vi "UI_(01)_Set_startup_controls_state.vi"(3 "error in (no error)":errorcluster, 4 "Settings cluster in":T3={"Defaults"={"Default User"=0.0, "VISA Resource Name "="", "Histogram parameters"={"max"=300.0, "min"=0.0, "# bins"=10, "threshold"=8.0, "thr. type"=enum."higher accepted"}}, "Recording and saving"={"Researcher name"="", "Name prefix"="", "Data post-processing"={"Filter type"=enum."Savitzky-Golay", "Length"=31, "Order"=3}, "Stop at"=0.0, "\"Stop at\" enabled"=FALSE, "Default save folder path"=path "", "Acquisition FPS"=enum."Max"}, "Geometry"={"Sensor board size"=enum."", "Bridge swap"=FALSE, "Twisted neck"=FALSE, "Bridge H. offset"=0.0, "Bridge V. offset"=0.0, "Magnets orientation"=0.0, "Cage type"=0, "Cage parameters"={"Round"=variant(i16 0), "Square"=variant(u16 0), "Donut-maze"=variant(u16 0), "T-maze"=variant(u8 0), "Sociability-maze"=variant(u8 0)}}, "IO parameters"={"IO general config."=0, "IO 1 configuration"=0, "IO 2 configuration"=0, "IO 3 configuration"=0, "IO 4 configuration"=0, "Activate ext. RS-232"=0, "IO inversion config."=0, "Sync capability"=1}, "Conditions presets array"=[{"Enabled"=FALSE, "Name"="", "Specifier(s)"=[], "Response"={"Response type"=enum."Air puff", "TTL port"=enum."Port 1", "TTL pulse length, ms"=0.0}, "Has been set"=FALSE}, {"Enabled"=FALSE, "Name"="", "Specifier(s)"=[], "Response"={"Response type"=enum."Air puff", "TTL port"=enum."Port 1", "TTL pulse length, ms"=0.0}, "Has been set"=FALSE}, {"Enabled"=FALSE, "Name"="", "Specifier(s)"=[], "Response"={"Response type"=enum."Air puff", "TTL port"=enum."Port 1", "TTL pulse length, ms"=0.0}, "Has been set"=FALSE}, {"Enabled"=FALSE, "Name"="", "Specifier(s)"=[], "Response"={"Response type"=enum."Air puff", "TTL port"=enum."Port 1", "TTL pulse length, ms"=0.0}, "Has been set"=FALSE}, {"Enabled"=FALSE, "Name"="", "Specifier(s)"=[], "Response"={"Response type"=enum."Air puff", "TTL port"=enum."Port 1", "TTL pulse length, ms"=0.0}, "Has been set"=FALSE}, {"Enabled"=FALSE, "Name"="", "Specifier(s)"=[], "Response"={"Response type"=enum."Air puff", "TTL port"=enum."Port 1", "TTL pulse length, ms"=0.0}, "Has been set"=FALSE}, {"Enabled"=FALSE, "Name"="", "Specifier(s)"=[], "Response"={"Response type"=enum."Air puff", "TTL port"=enum."Port 1", "TTL pulse length, ms"=0.0}, "Has been set"=FALSE}, {"Enabled"=FALSE, "Name"="", "Specifier(s)"=[], "Response"={"Response type"=enum."Air puff", "TTL port"=enum."Port 1", "TTL pulse length, ms"=0.0}, "Has been set"=FALSE}, {"Enabled"=FALSE, "Name"="", "Specifier(s)"=[], "Response"={"Response type"=enum."Air puff", "TTL port"=enum."Port 1", "TTL pulse length, ms"=0.0}, "Has been set"=FALSE}, {"Enabled"=FALSE, "Name"="", "Specifier(s)"=[], "Response"={"Response type"=enum."Air puff", "TTL port"=enum."Port 1", "TTL pulse length, ms"=0.0}, "Has been set"=FALSE}, {"Enabled"=FALSE, "Name"="", "Specifier(s)"=[], "Response"={"Response type"=enum."Air puff", "TTL port"=enum."Port 1", "TTL pulse length, ms"=0.0}, "Has been set"=FALSE}, {"Enabled"=FALSE, "Name"="", "Specifier(s)"=[], "Response"={"Response type"=enum."Air puff", "TTL port"=enum."Port 1", "TTL pulse length, ms"=0.0}, "Has been set"=FALSE}, {"Enabled"=FALSE, "Name"="", "Specifier(s)"=[], "Response"={"Response type"=enum."Air puff", "TTL port"=enum."Port 1", "TTL pulse length, ms"=0.0}, "Has been set"=FALSE}, {"Enabled"=FALSE, "Name"="", "Specifier(s)"=[], "Response"={"Response type"=enum."Air puff", "TTL port"=enum."Port 1", "TTL pulse length, ms"=0.0}, "Has been set"=FALSE}], "Calibration parameters"={"Timing calibration sw/hw"=1.0, "True FPS"=80.0, "True frame time, s"=80.0, "Disp. calibration info"=[]}} {"Calibration parameters"."True frame time, s" format="%.10g"; "Calibration parameters"."Disp. calibration info"."Speed, µl per ms" format="%.3g"; "Calibration parameters"."True FPS" format="%.10g"; "Calibration parameters"."Timing calibration sw/hw" format="%.10g"; "Conditions presets array"."Specifier(s)"."Validity criteria(s)"."Validity value" min=0.0 step=0.1 format="%.2g"; "Conditions presets array"."Specifier(s)"."Value" step=1.0 format="%#.2g"; "Recording and saving"."Data post-processing"."Order" min=3 max=11 step=2; "Recording and saving"."Data post-processing"."Length" min=5 max=301 step=2; "Geometry"."Cage type" items=["Round", "Square", "Donut-maze", "T-maze", "Sociability maze", ""]}, 5 "All UI references in":T24) -> (0 "error out":errorcluster)   [LabVIEW 2018, in "Tracker Main.lvlib"]
uses:
  Tracker Main.lvlib
  Common/Typedefs/CTL_All_UI_References_2.ctl
  Common/Typedefs/CTL_Panes_and_VIs_References.ctl
  Common/Typedefs/CTL_Indicators_References_2.ctl
  Common/Typedefs/CTL_Controls_References_2.ctl
  SubVi's/Controls/CTL_Histogram_Properties.ctl
  <vilib>/Utility/miscctls.llb/LVRangeTypeDef.ctl
  Common/Typedefs/CTL_Settings_cluster_2.ctl
  SubVi's/Controls/CTL_Histogram_parameters.ctl
  SubVi's/Controls/CTL_Filter_selector.ctl
  SubVi's/Controls/CTL_Acquisition_speed_selector.ctl
  Common/Typedefs/CTL_Segmented_plot_parameters_2.ctl
  Cage Diagram/Typedefs/CTL_Cage_type.ctl
  SubVi's/Controls/CTL_Cage_all_segmentation_params_set.ctl
  SubVi's/Controls/CTL_IO_params_cluster.ctl
  SubVi's/Controls/CTL_Conditions_Array.ctl
  SubVi's/Controls/CTL_Conditions_Cluster.ctl
  SubVi's/Controls/CTL_Condition_type.ctl
  SubVi's/Controls/CTL_Comparison_type.ctl
  SubVi's/Controls/CTL_Validity_check_criteria.ctl
  SubVi's/Controls/CTL_Response_info.ctl
  SubVi's/Controls/CTL_Condition_response_type.ctl
  SubVi's/Controls/CTL_Reponse_port_info.ctl
  SubVi's/Controls/CTL_Calibration_parameters.ctl
  SubVi's/Controls/CTL_Dispenser_calibration_info.ctl
  <vilib>/Utility/miscctls.llb/LVPointTypeDef.ctl
  Common/Typedefs/CTL_IO_Ports_activity_indicator.ctl
  <vilib>/Utility/error.llb/Error Cluster From Error Code.vi
  <vilib>/ErrorRing/Error Ring.xnode
  Common_Resources.lvlib
  Cage Diagram/Cage Diagram.lvlib
panel:
  out "Controls References":T1
  out "Indicators References":T2
  in  "Histogram initialization cluster":T21={"X Scale.Range"={"Minimum"=0.0, "Maximum"=13.0, "Increment"=1.0, "Minor Increment"=1.0, "Start"=0.0}, "Caption.Text"="Zone preference (normalized)", "X Scale.Offset and Multiplier:Multiplier"=1.0, "X Scale.Offset and Multiplier:Offset"=0.0, "X Scale.Scale Fit"=2, "X Scale.Display Format:Precision"=0, "Y Scale.Mapping Mode"=0, "Zones preference empty initialized array"=[0, 0, 0, 0, 0, 0, 0, 0, 0, 0, 0, 0, 0, 0], "Plot.Fill/Point Color"=15790320}
  out "Panes references":T23
  out "Controls references params":string[][](array[string])
  out "Indicators references params":string[][](array[string])
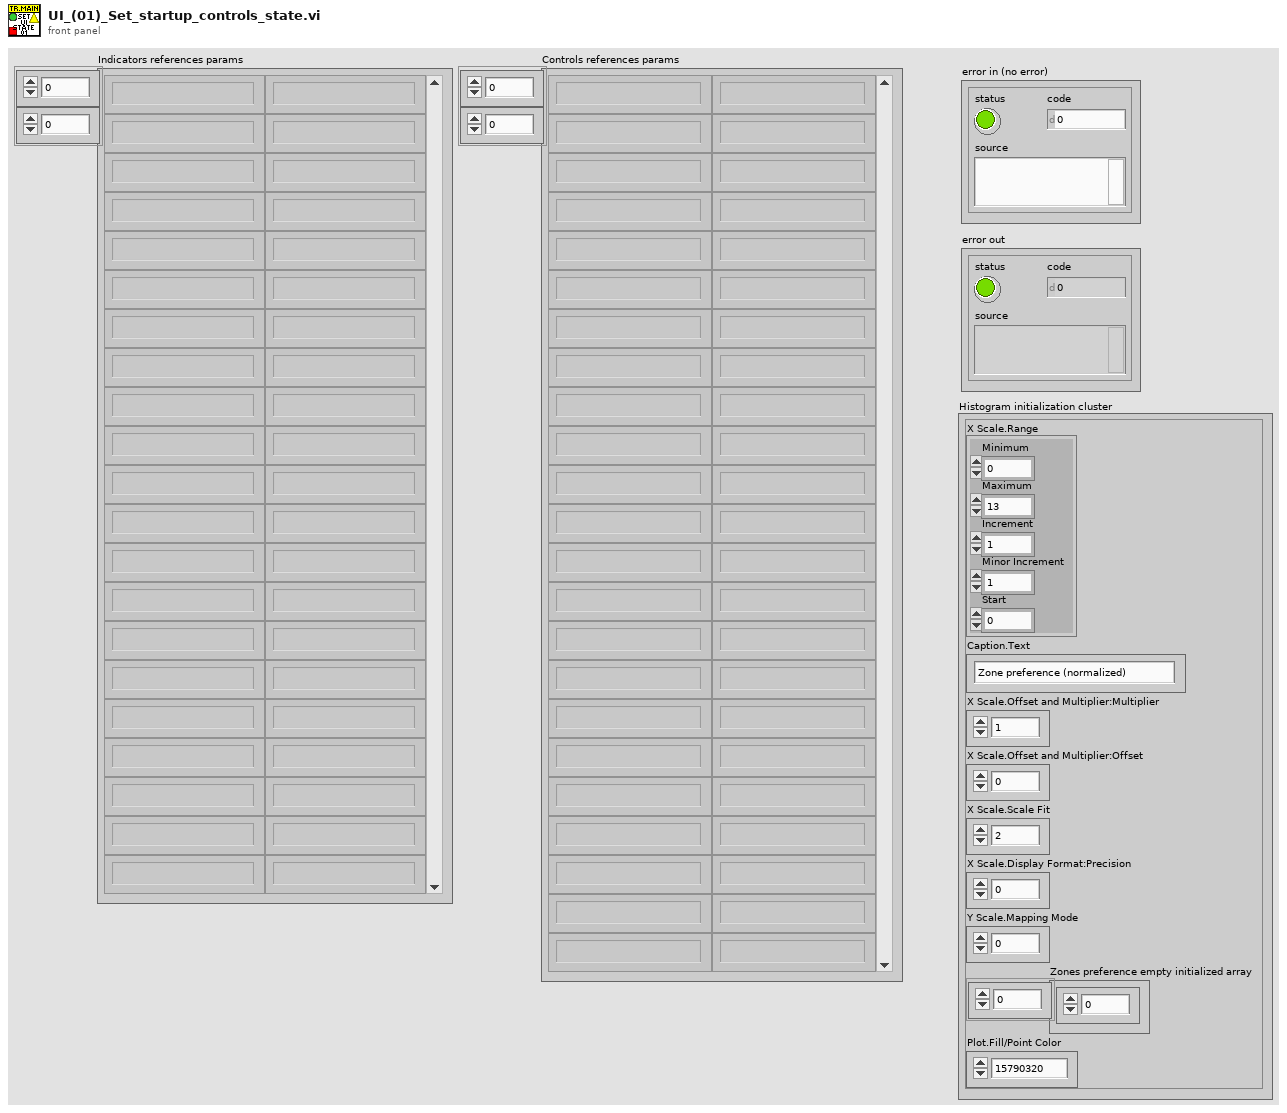
[diagram p1: front panel]
types:
  T1 = typedef "Common_Resources.lvlib/CTL_Controls_References_2.ctl" = cluster{"Timeline":refnum<vi>, "Play/Pause":refnum<vi>, "Record/Stop":refnum<vi>, "Exact time pos.":refnum<vi>, "Add Reward":refnum<vi>, "Modify Reward":refnum<vi>, "Remove Reward":refnum<vi>, "Show zones":refnum<vi>, "Show magnets":refnum<vi>, "Rainbow (time)":refnum<vi>, "Rainbow (speed)":refnum<vi>, "Show heatmap":refnum<vi>, "Show full track":refnum<vi>, "Playback speed":refnum<vi>, "Trace, s":refnum<vi>, "Set/Rec and Analyse Tab":refnum<vi>, "Reward and stimulation":refnum<vi>, "Speed threshold":refnum<vi>, "Multiplyer of chart RX":refnum<vi>, "Reset barplot":refnum<vi>, "Open File":refnum<vi>, "Start over":refnum<vi>}
  T2 = typedef "Common_Resources.lvlib/CTL_Indicators_References_2.ctl" = cluster{"HW info":refnum<vi>, "Port":refnum<vi>, "Cage size":refnum<vi>, "Current zone":refnum<vi>, "Current Time":refnum<vi>, "Since track start":refnum<vi>, "Key_pressed":refnum<vi>, "Status":refnum<vi>, "Status History":refnum<vi>, "IO status":refnum<vi>, "Ports Activity":refnum<vi>, "Active rules":refnum<vi>, "Histograms":refnum<vi>, "Mouse speed":refnum<vi>, "Mouse speed, mm/s":refnum<vi>, "Average speed, mm/s":refnum<vi>, "Run distance, m":refnum<vi>, "Running, perc. of time":refnum<vi>, "CPU load":refnum<vi>, "Diagram ref":refnum<vi>}
  T3 = typedef "Common_Resources.lvlib/CTL_Settings_cluster_2.ctl" = cluster{"Defaults":cluster{"Default User":dbl, "VISA Resource Name ":string, "Histogram parameters":T4}, "Recording and saving":cluster{"Researcher name":string, "Name prefix":string, "Data post-processing":T5, "Stop at":dbl, "\"Stop at\" enabled":bool, "Default save folder path":path, "Acquisition FPS":T6}, "Geometry":T7, "IO parameters":T10, "Conditions presets array":T11, "Calibration parameters":T19}
  T4 = typedef "Common_Resources.lvlib/CTL_Histogram_parameters.ctl" = cluster{"max":dbl, "min":dbl, "# bins":i32, "threshold":dbl, "thr. type":enum16{"higher accepted", "lower accepted"}}
  T5 = typedef "Common_Resources.lvlib/CTL_Filter_selector.ctl" = cluster{"Filter type":enum16{"None", "Savitzky-Golay"}, "Length":i32, "Order":i32}
  T6 = typedef "Common_Resources.lvlib/CTL_Acquisition_speed_selector.ctl" = enum16{"Max", "Optimal", "Eco"}
  T7 = typedef "Common_Resources.lvlib/CTL_Segmented_plot_parameters_2.ctl" = cluster{"Sensor board size":enum16{"", "Large"}, "Bridge swap":bool, "Twisted neck":bool, "Bridge H. offset":sgl, "Bridge V. offset":sgl, "Magnets orientation":sgl, "Cage type":T8, "Cage parameters":T9}
  T8 = typedef "Cage Diagram.lvlib/CTL_Cage_type.ctl" = u16
  T9 = typedef "Common_Resources.lvlib/CTL_Cage_all_segmentation_params_set.ctl" = cluster{"Round":variant, "Square":variant, "Donut-maze":variant, "T-maze":variant, "Sociability-maze":variant}
  T10 = typedef "Common_Resources.lvlib/CTL_IO_params_cluster.ctl" = cluster{"IO general config.":u16, "IO 1 configuration":u16, "IO 2 configuration":u16, "IO 3 configuration":u16, "IO 4 configuration":u16, "Activate ext. RS-232":u16, "IO inversion config.":u16, "Sync capability":u8}
  T11 = typedef "Common_Resources.lvlib/CTL_Conditions_Array.ctl" = T12[]
  T12 = typedef "Common_Resources.lvlib/CTL_Conditions_Cluster.ctl" = cluster{"Enabled":bool, "Name":string, "Specifier(s)":cluster{"Specifier enabled":bool, "Condition type":T13, "Comparison type":T14, "Value":dbl, "Validity criteria(s)":cluster{"V. check enabled":bool, "Criteria":T15, "Validity value":dbl}[]}[], "Response":T16, "Has been set":bool}
  T13 = typedef "Common_Resources.lvlib/CTL_Condition_type.ctl" = enum16{"Speed", "Zone", "Angle to wall"}
  T14 = typedef "Common_Resources.lvlib/CTL_Comparison_type.ctl" = enum16{"Less", "Less or Equal", "Equal", "Greater or Equal", "Greater", "Not Equal"}
  T15 = typedef "Common_Resources.lvlib/CTL_Validity_check_criteria.ctl" = enum16{"Running bout (seconds)", "Running bout (meters)"}
  T16 = typedef "Common_Resources.lvlib/CTL_Response_info.ctl" = cluster{"Response type":T17, "TTL port":T18, "TTL pulse length, ms":dbl}
  T17 = typedef "Common_Resources.lvlib/CTL_Condition_response_type.ctl" = enum16{"None", "Air puff", "Liquid reward", "TTL pulse", "TTL pulse (ubr)", "TTL signal"}
  T18 = typedef "Common_Resources.lvlib/CTL_Reponse_port_info.ctl" = enum16{"Port 1", "Port 2", "Port 3", "Port 4"}
  T19 = typedef "Common_Resources.lvlib/CTL_Calibration_parameters.ctl" = cluster{"Timing calibration sw/hw":dbl, "True FPS":dbl, "True frame time, s":dbl, "Disp. calibration info":T20}
  T20 = typedef "Common_Resources.lvlib/CTL_Dispenser_calibration_info.ctl" = cluster{"Channel":u8, "Speed, µl per ms":dbl}[]
  T21 = typedef "Common_Resources.lvlib/CTL_Histogram_Properties.ctl" = cluster{"X Scale.Range":T22, "Caption.Text":string, "X Scale.Offset and Multiplier:Multiplier":dbl, "X Scale.Offset and Multiplier:Offset":dbl, "X Scale.Scale Fit":u8, "X Scale.Display Format:Precision":u8, "Y Scale.Mapping Mode":u8, "Zones preference empty initialized array":i32[], "Plot.Fill/Point Color":u32}
  T22 = typedef "LVRangeTypeDef.ctl" = cluster{"Minimum":dbl, "Maximum":dbl, "Increment":dbl, "Minor Increment":dbl, "Start":dbl}
  T23 = typedef "Common_Resources.lvlib/CTL_Panes_and_VIs_References.ctl" = cluster{"Pane":refnum<vi>, "This VI":refnum<vi>, "Menu":refnum<k9>}
  T24 = typedef "Common_Resources.lvlib/CTL_All_UI_References_2.ctl" = cluster{"Service references":T23, "Indicators References":T2, "Controls References":T1}
  T25 = typedef "LVPointTypeDef.ctl" = cluster{"Horizontal":i16, "Vertical":i16}
  T26 = typedef "Common_Resources.lvlib/CTL_IO_Ports_activity_indicator.ctl" = cluster{"IO1 act":bool, "IO2 act":bool, "IO3 act":bool, "IO4 act":bool}
  T27 = cluster{"01":bool, "02":bool, "03":bool, "04":bool, "05":bool, "06":bool, "07":bool, "08":bool, "09":bool}
  T28 = enum8{"Enabled", "Disabled", "Disabled and Grayed Out"}
  T29 = enum32{"Page Enabled", "Page Disabled", "Page Disabled & Grayed"}
  T30 = cluster{"Slider":dbl, "Slider":dbl, "Slider":dbl}
  T31 = typedef "Common_Resources.lvlib/CTL_IO_status_indicator_2.ctl" = cluster{"IO1":bool, "IO2":bool, "IO3":bool, "IO4":bool, "St1":bool, "St2":bool, "St3":bool, "St4":bool, "Ext1":bool, "Ext2":bool, "Ext3":bool, "Ext4":bool, "Syn1":bool, "Syn2":bool, "Syn3":bool, "Syn4":bool}
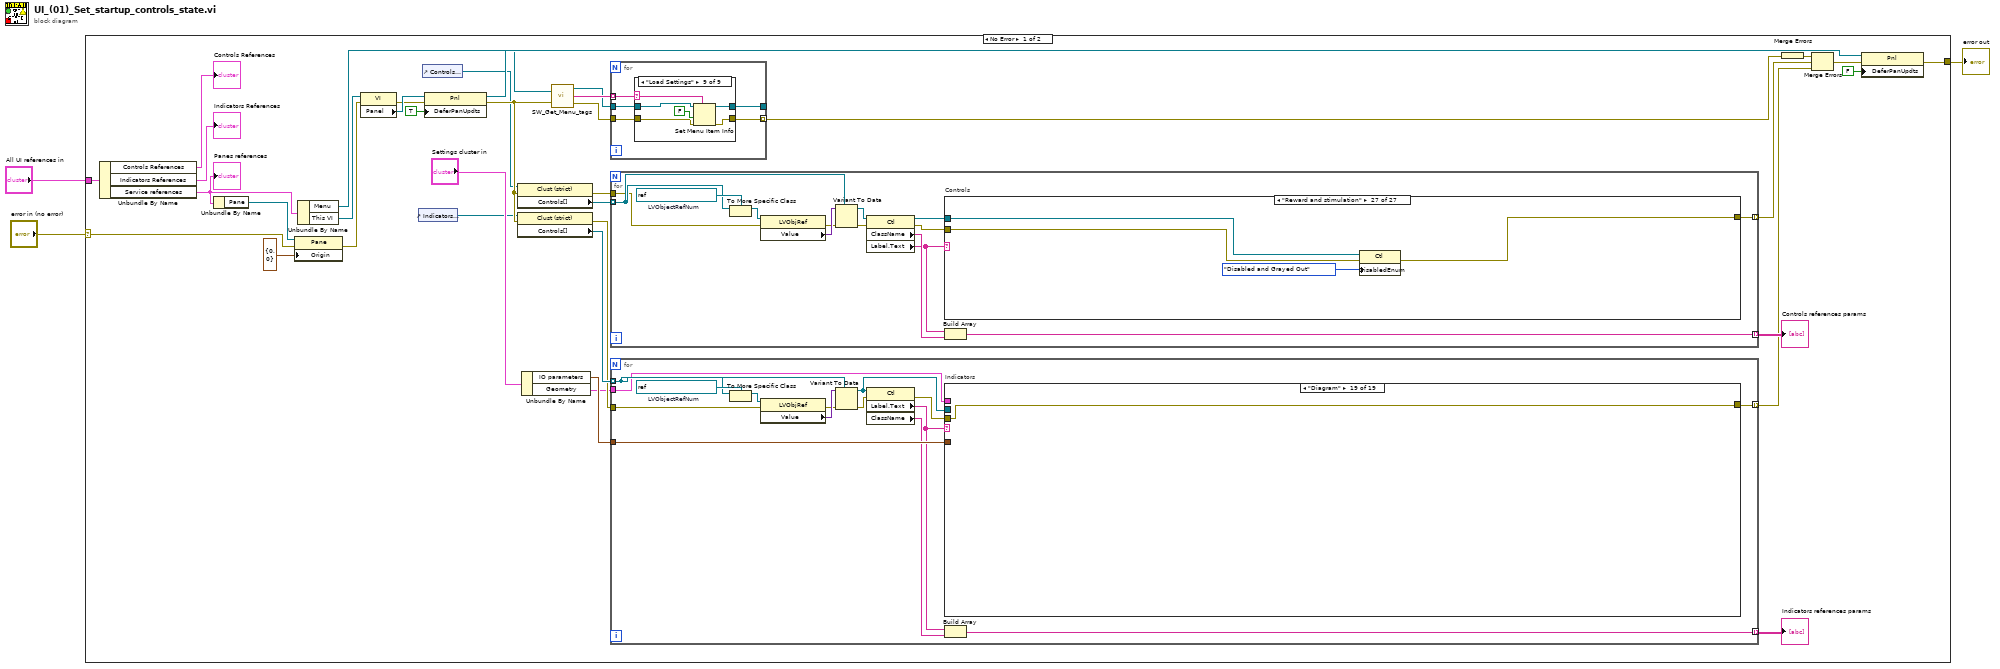
[diagram p0: block diagram]
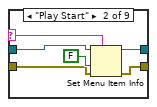
[diagram p3: hidden frame]
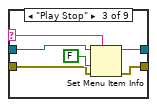
[diagram p4: hidden frame]
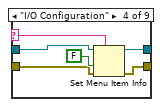
[diagram p5: hidden frame]
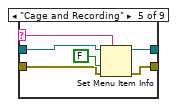
[diagram p6: hidden frame]
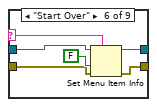
[diagram p7: hidden frame]
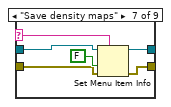
[diagram p8: hidden frame]
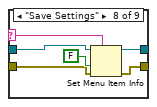
[diagram p9: hidden frame]
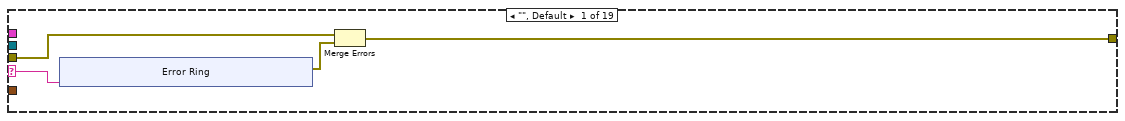
[diagram p10: hidden frame]
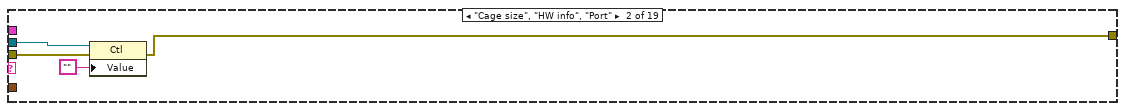
[diagram p11: hidden frame]
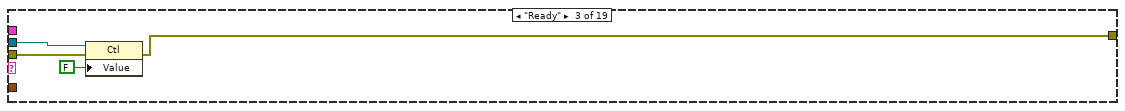
[diagram p12: hidden frame]
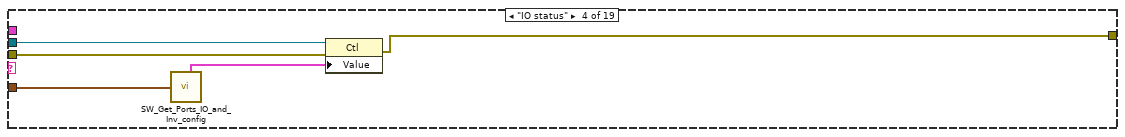
[diagram p13: hidden frame]
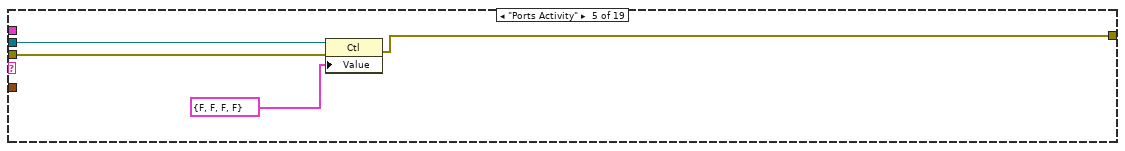
[diagram p14: hidden frame]
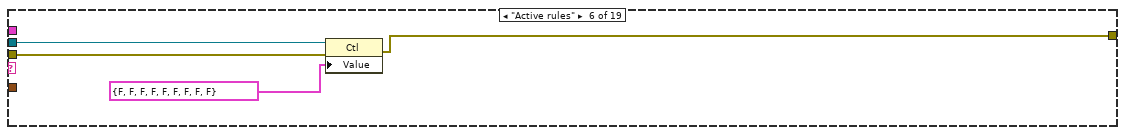
[diagram p15: hidden frame]
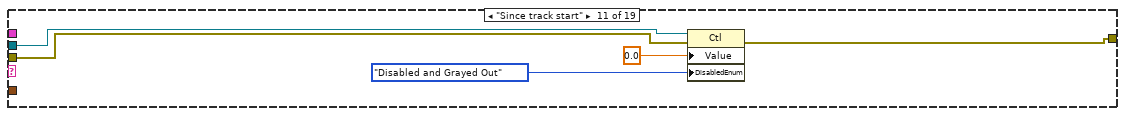
[diagram p20: hidden frame]
diagram:
  n1 = case shown="No Error" "error in (no error)" {
    selector: "error in (no error)" -> [w4 w435]
    tunnel: "All UI references in" -> [w39 _]
    tunnel: [w24 w435] -> w2
    frame No Error {
      n2 = Unbundle By Name(w39) -> ("Controls References"=→"Controls References":T1, "Indicators References"=→"Indicators References":T2, "Service references"=w9:T23)
      "Panes references" <- w9
      n3 = Unbundle By Name(w9) -> ("Pane"=w21:refnum<vi>)
      n4 = property class="Pane"(reference=w21, error in=w4, "Origin"=T25 {"Horizontal"=0, "Vertical"=0}) -> (error out=w20:errorcluster)  [unwired: 1 out]
      n5 = Unbundle By Name(w9) -> ("Menu"=w18:refnum<k9>, "This VI"=w32:refnum<vi>)
      n6 = property class="VI"(reference=w32, error in=w20) -> (error out=w25:errorcluster, "Panel"=w34:refnum<vi>)  [unwired: 1 out]
      n7 = control-ref of="Indicators References"() -> (w7:refnum<vi>)
      n8 = control-ref of="Controls References"() -> (w5:refnum<vi>)
      n9 = property class="Pnl"(reference=w34, error in=w25, "DeferPanUpdts"=TRUE ("Defer Panel Updates")) -> (reference out=w26:refnum<vi>, error out=w17:errorcluster)
      n10 = property class="Clust (strict)"(reference=w5, error in=w17) -> (error out=w31:errorcluster, "Controls[]"=w38:refnum<vi>[])  [unwired: 1 out]
      n11 = property class="Clust (strict)"(reference=w7, error in=w17) -> (error out=w30:errorcluster, "Controls[]"=w37:refnum<vi>[])  [unwired: 1 out]
      n12 = Unbundle By Name("Settings cluster in") -> ("IO parameters"=w22:T10, "Geometry"=w10:T7)
      n13 = call "SW_Get_Menu_tags.vi"("Menu ref in"=w18, "error in (no error)"=w17) -> ("Menu ref out"=w14:refnum<k9>, "(Sub)menu tags"=w16:string[], "error out"=w15:errorcluster)
      n14 = for {
        tunnel: w16 -> [w44] mode=indexing
        tunnel: w15 -> [w43]
        tunnel: [w42] -> w13 mode=indexing
        tunnel: [w41] -> _
        tunnel: w14 -> [w40]
        n15 = case shown="\"Load Settings\"" w44 {
          selector: w44 -> [_ w52 w58 w64 w70 w76 w82 w88 w94]
          tunnel: w43 -> [w46 w50 w56 w62 w68 w74 w80 w86 w92]
          tunnel: [w46 w49 w55 w61 w67 w73 w79 w85 w91] -> w42
          tunnel: [w45 w48 w54 w60 w66 w72 w78 w84 w90] -> w41
          tunnel: w40 -> [w45 w47 w53 w59 w65 w71 w77 w83 w89]
          frame "", Default {
          }
          frame "Play Start" {
            n16 = Set Menu Item Info(7:w52, 8:w50, 9:FALSE ("enabled"), 11:w47) -> (0:w49:errorcluster, 3:w48:refnum<k9>)  [unwired: 3 in]
          }
          frame "Play Stop" {
            n17 = Set Menu Item Info(7:w58, 8:w56, 9:FALSE ("enabled"), 11:w53) -> (0:w55:errorcluster, 3:w54:refnum<k9>)  [unwired: 3 in]
          }
          frame "I/O Configuration" {
            n18 = Set Menu Item Info(7:w64, 8:w62, 9:FALSE ("enabled"), 11:w59) -> (0:w61:errorcluster, 3:w60:refnum<k9>)  [unwired: 3 in]
          }
          frame "Cage and Recording" {
            n19 = Set Menu Item Info(7:w70, 8:w68, 9:FALSE ("enabled"), 11:w65) -> (0:w67:errorcluster, 3:w66:refnum<k9>)  [unwired: 3 in]
          }
          frame "Start Over" {
            n20 = Set Menu Item Info(7:w76, 8:w74, 9:FALSE ("enabled"), 11:w71) -> (0:w73:errorcluster, 3:w72:refnum<k9>)  [unwired: 3 in]
          }
          frame "Save density maps" {
            n21 = Set Menu Item Info(7:w82, 8:w80, 9:FALSE ("enabled"), 11:w77) -> (0:w79:errorcluster, 3:w78:refnum<k9>)  [unwired: 3 in]
          }
          frame "Save Settings" {
            n22 = Set Menu Item Info(7:w88, 8:w86, 9:FALSE ("enabled"), 11:w83) -> (0:w85:errorcluster, 3:w84:refnum<k9>)  [unwired: 3 in]
          }
          frame "Load Settings" {
            n23 = Set Menu Item Info(7:w94, 8:w92, 9:FALSE ("enabled"), 11:w89) -> (0:w91:errorcluster, 3:w90:refnum<k9>)  [unwired: 3 in]
          }
        }
      }
      n24 = for {
        tunnel: w38 -> [w202] mode=indexing
        tunnel: [w199] -> w35 mode=indexing
        tunnel: w31 -> [w198]
        tunnel: [w194] -> w23 mode=indexing
        w204 = refnum<vi> refnum  # LVObjectRefNum
        n25 = To More Specific Class(target class=w204, reference=w202) -> (specific class reference=w205:refnum<vi>)  [unwired: 1 in, 1 out]
        n26 = property class="LVObjRef"(reference=w205, error in=w198) -> (error out=w197:errorcluster, "Value"=w203:variant)  [unwired: 1 out]
        n27 = Variant To Data(error in=w197, type=w202, Variant=w203) -> (data=w201:refnum<vi>, error out=w196:errorcluster)
        n28 = property class="Ctl"(reference=w201, error in=w196) -> (reference out=w192:refnum<vi>, error out=w193:errorcluster, "ClassName"=w200:string, "Label.Text"=w195:string)
        n29 = case "Controls" shown="\"Reward and stimulation\"" w195 {
          selector: w195 -> [w206 _ _ _ _ _ _ _ _ _ _ _ _ _ _ _ _ _ _ _ _ _ _ _ _ _ _]
          tunnel: [w208 w222 w224 w240 w248 w256 w264 w272 w281 w290 w298 w306 w314 w322 w330 w338 w346 w354 w362 w370 w378 w385 w392 w400 w416 w425 w431] -> w194
          tunnel: w193 -> [w209 w221 w228 w242 w250 w258 w266 w274 w283 w292 w300 w308 w316 w324 w332 w340 w348 w356 w364 w372 w380 w387 w394 w402 w418 w427 w432]
          tunnel: w192 -> [_ w219 w233 w245 w253 w261 w269 w277 w286 w295 w303 w311 w319 w327 w335 w343 w351 w359 w367 w375 w383 w390 w397 w405 w421 w430 w433]
          frame "", Default {
            n30 = xnode "Error Ring"("parameter 0"=w206) -> ("error out"=w207:errorcluster)
            n31 = Merge Errors(w209, w207) -> (w208:errorcluster)
          }
          frame "Cage radial segmentation" {
            w217 = refnum<vi> refnum  # Cluster
            n32 = To More Specific Class(target class=w217, reference=w219, error in=w221) -> (specific class reference=w218:refnum<vi>, error out=w220:errorcluster)
            n33 = property class="Clust"(reference=w218, error in=w220, "DisabledEnum"=T28."Disabled and Grayed Out" ("Disabled")) -> (error out=w222:errorcluster)  [unwired: 1 out]
          }
          frame "Set/Rec and Analyse Tab" {
            w230 = refnum<vi> refnum  # TabControl
            n34 = To More Specific Class(target class=w230, reference=w233, error in=w228) -> (specific class reference=w231:refnum<vi>, error out=w227:errorcluster)
            n35 = property class="TabCtl"(reference=w231, error in=w227, "Value"=enum32{"Settings", "Recording and Analysis"}."Settings") -> (error out=w226:errorcluster, "Pages"=w229:refnum<vi>[])  [unwired: 1 out]
            n36 = for {
              tunnel: w229 -> [w236] mode=indexing
              tunnel: w226 -> [w235]
              tunnel: [w234] -> w225 mode=indexing
              n37 = property class="Page"(reference=w236, error in=w235, "PageEnb"=T29."Page Disabled & Grayed" ("Page Enabled State")) -> (error out=w234:errorcluster)  [unwired: 1 out]
            }
            n38 = Merge Errors(w225) -> (w224:errorcluster)
          }
          frame "Check HW connection" {
            w244 = refnum<vi> refnum  # Boolean
            n39 = To More Specific Class(target class=w244, reference=w245, error in=w242) -> (specific class reference=w243:refnum<vi>, error out=w241:errorcluster)
            n40 = property class="Bool"(reference=w243, error in=w241, "Value"=FALSE, "DisabledEnum"=T28."Disabled and Grayed Out" ("Disabled")) -> (error out=w240:errorcluster)  [unwired: 1 out]
          }
          frame "Save settings" {
            w252 = refnum<vi> refnum  # Boolean
            n41 = To More Specific Class(target class=w252, reference=w253, error in=w250) -> (specific class reference=w251:refnum<vi>, error out=w249:errorcluster)
            n42 = property class="Bool"(reference=w251, error in=w249, "Value"=FALSE, "DisabledEnum"=T28."Disabled and Grayed Out" ("Disabled")) -> (error out=w248:errorcluster)  [unwired: 1 out]
          }
          frame "Set IO config" {
            w260 = refnum<vi> refnum  # Boolean
            n43 = To More Specific Class(target class=w260, reference=w261, error in=w258) -> (specific class reference=w259:refnum<vi>, error out=w257:errorcluster)
            n44 = property class="Bool"(reference=w259, error in=w257, "Value"=FALSE, "DisabledEnum"=T28."Disabled and Grayed Out" ("Disabled")) -> (error out=w256:errorcluster)  [unwired: 1 out]
          }
          frame "Reset zones" {
            w268 = refnum<vi> refnum  # Boolean
            n45 = To More Specific Class(target class=w268, reference=w269, error in=w266) -> (specific class reference=w267:refnum<vi>, error out=w265:errorcluster)
            n46 = property class="Bool"(reference=w267, error in=w265, "Value"=FALSE, "DisabledEnum"=T28."Disabled and Grayed Out" ("Disabled")) -> (error out=w264:errorcluster)  [unwired: 1 out]
          }
          frame "Reset stimuli" {
            w276 = refnum<vi> refnum  # Boolean
            n47 = To More Specific Class(target class=w276, reference=w277, error in=w274) -> (specific class reference=w275:refnum<vi>, error out=w273:errorcluster)
            n48 = property class="Bool"(reference=w275, error in=w273, "Value"=FALSE, "DisabledEnum"=T28."Disabled and Grayed Out" ("Disabled")) -> (error out=w272:errorcluster)  [unwired: 1 out]
          }
          frame "Record/Stop" {
            w285 = refnum<vi> refnum  # Boolean
            n49 = To More Specific Class(target class=w285, reference=w286, error in=w283) -> (specific class reference=w284:refnum<vi>, error out=w282:errorcluster)
            n50 = property class="Bool"(reference=w284, error in=w282, "Value"=FALSE, "DisabledEnum"=T28."Disabled and Grayed Out" ("Disabled"), "Visible"=TRUE) -> (error out=w281:errorcluster)  [unwired: 1 out]
          }
          frame "Start over" {
            w294 = refnum<vi> refnum  # Boolean
            n51 = To More Specific Class(target class=w294, reference=w295, error in=w292) -> (specific class reference=w293:refnum<vi>, error out=w291:errorcluster)
            n52 = property class="Bool"(reference=w293, error in=w291, "Value"=FALSE, "DisabledEnum"=T28."Disabled and Grayed Out" ("Disabled"), "Visible"=FALSE) -> (error out=w290:errorcluster)  [unwired: 1 out]
          }
          frame "Reset barplot" {
            w302 = refnum<vi> refnum  # Boolean
            n53 = To More Specific Class(target class=w302, reference=w303, error in=w300) -> (specific class reference=w301:refnum<vi>, error out=w299:errorcluster)
            n54 = property class="Bool"(reference=w301, error in=w299, "Value"=FALSE, "DisabledEnum"=T28."Disabled and Grayed Out" ("Disabled")) -> (error out=w298:errorcluster)  [unwired: 1 out]
          }
          frame "Multiplyer of chart RX" {
            w310 = refnum<vi> refnum  # Slide
            n55 = To More Specific Class(target class=w310, reference=w311, error in=w308) -> (specific class reference=w309:refnum<vi>, error out=w307:errorcluster)
            n56 = property class="Slide"(reference=w309, error in=w307, "Value"=u8 1, "DisabledEnum"=T28."Disabled and Grayed Out" ("Disabled")) -> (error out=w306:errorcluster)  [unwired: 1 out]
          }
          frame "Show zones" {
            w318 = refnum<vi> refnum  # Boolean
            n57 = To More Specific Class(target class=w318, reference=w319, error in=w316) -> (specific class reference=w317:refnum<vi>, error out=w315:errorcluster)
            n58 = property class="Bool"(reference=w317, error in=w315, "Value"=TRUE, "DisabledEnum"=T28."Disabled and Grayed Out" ("Disabled")) -> (error out=w314:errorcluster)  [unwired: 1 out]
          }
          frame "Show magnets" {
            w326 = refnum<vi> refnum  # Boolean
            n59 = To More Specific Class(target class=w326, reference=w327, error in=w324) -> (specific class reference=w325:refnum<vi>, error out=w323:errorcluster)
            n60 = property class="Bool"(reference=w325, error in=w323, "Value"=TRUE, "DisabledEnum"=T28."Disabled and Grayed Out" ("Disabled")) -> (error out=w322:errorcluster)  [unwired: 1 out]
          }
          frame "Rainbow (speed)", "Rainbow (time)" {
            w334 = refnum<vi> refnum  # Boolean
            n61 = To More Specific Class(target class=w334, reference=w335, error in=w332) -> (specific class reference=w333:refnum<vi>, error out=w331:errorcluster)
            n62 = property class="Bool"(reference=w333, error in=w331, "Value"=FALSE, "DisabledEnum"=T28."Disabled and Grayed Out" ("Disabled")) -> (error out=w330:errorcluster)  [unwired: 1 out]
          }
          frame "Add Reward", "Modify Reward", "Remove Reward" {
            w342 = refnum<vi> refnum  # Boolean
            n63 = To More Specific Class(target class=w342, reference=w343, error in=w340) -> (specific class reference=w341:refnum<vi>, error out=w339:errorcluster)
            n64 = property class="Bool"(reference=w341, error in=w339, "Value"=FALSE, "DisabledEnum"=T28."Disabled and Grayed Out" ("Disabled")) -> (error out=w338:errorcluster)  [unwired: 1 out]
          }
          frame "Show heatmap" {
            w350 = refnum<vi> refnum  # Boolean
            n65 = To More Specific Class(target class=w350, reference=w351, error in=w348) -> (specific class reference=w349:refnum<vi>, error out=w347:errorcluster)
            n66 = property class="Bool"(reference=w349, error in=w347, "Value"=FALSE, "DisabledEnum"=T28."Disabled and Grayed Out" ("Disabled")) -> (error out=w346:errorcluster)  [unwired: 1 out]
          }
          frame "Show full track" {
            w358 = refnum<vi> refnum  # Boolean
            n67 = To More Specific Class(target class=w358, reference=w359, error in=w356) -> (specific class reference=w357:refnum<vi>, error out=w355:errorcluster)
            n68 = property class="Bool"(reference=w357, error in=w355, "Value"=FALSE, "DisabledEnum"=T28."Disabled and Grayed Out" ("Disabled")) -> (error out=w354:errorcluster)  [unwired: 1 out]
          }
          frame "Open File" {
            w366 = refnum<vi> refnum  # Boolean
            n69 = To More Specific Class(target class=w366, reference=w367, error in=w364) -> (specific class reference=w365:refnum<vi>, error out=w363:errorcluster)
            n70 = property class="Bool"(reference=w365, error in=w363, "Value"=FALSE, "DisabledEnum"=T28."Disabled and Grayed Out" ("Disabled")) -> (error out=w362:errorcluster)  [unwired: 1 out]
          }
          frame "Play/Pause" {
            w374 = refnum<vi> refnum  # Boolean
            n71 = To More Specific Class(target class=w374, reference=w375, error in=w372) -> (specific class reference=w373:refnum<vi>, error out=w371:errorcluster)
            n72 = property class="Bool"(reference=w373, error in=w371, "Value"=FALSE, "DisabledEnum"=T28."Disabled and Grayed Out" ("Disabled")) -> (error out=w370:errorcluster)  [unwired: 1 out]
          }
          frame "Trace, s" {
            w382 = refnum<vi> refnum  # Slide
            n73 = To More Specific Class(target class=w382, reference=w383, error in=w380) -> (specific class reference=w381:refnum<vi>, error out=w379:errorcluster)
            n74 = property class="Slide"(reference=w381, error in=w379, "Value"=u8 5, "DisabledEnum"=T28."Disabled and Grayed Out" ("Disabled")) -> (error out=w378:errorcluster)  [unwired: 1 out]
          }
          frame "Speed threshold" {
            w389 = refnum<vi> refnum  # Digital
            n75 = To More Specific Class(target class=w389, reference=w390, error in=w387) -> (specific class reference=w388:refnum<vi>, error out=w386:errorcluster)
            n76 = property class="DigNum"(reference=w388, error in=w386, "DisabledEnum"=T28."Disabled and Grayed Out" ("Disabled")) -> (error out=w385:errorcluster)  [unwired: 1 out]
          }
          frame "Exact time pos." {
            w396 = refnum<vi> refnum  # Digital
            n77 = To More Specific Class(target class=w396, reference=w397, error in=w394) -> (specific class reference=w395:refnum<vi>, error out=w393:errorcluster)
            n78 = property class="DigNum"(reference=w395, error in=w393, "DisabledEnum"=T28."Disabled and Grayed Out" ("Disabled")) -> (error out=w392:errorcluster)  [unwired: 1 out]
          }
          frame "Playback speed" {
            w404 = refnum<vi> refnum  # Ring
            n79 = To More Specific Class(target class=w404, reference=w405, error in=w402) -> (specific class reference=w403:refnum<vi>, error out=w401:errorcluster)
            n80 = property class="Ring"(reference=w403, error in=w401, "Value"=u8 120, "DisabledEnum"=T28."Disabled and Grayed Out" ("Disabled")) -> (error out=w400:errorcluster)  [unwired: 1 out]
          }
          frame "Timeline" {
            w407 = 0.0 ("Slider")
            w420 = refnum<vi> refnum  # Slide
            n81 = To More Specific Class(target class=w420, reference=w421, error in=w418) -> (specific class reference=w419:refnum<vi>, error out=w417:errorcluster)
            n82 = Bundle(cluster=T30 {"Slider"=0.0, "Slider"=0.0, "Slider"=0.0} ("Timeline"), "Slider"=w407, "Slider"=0.001, "Slider"=w407) -> (w413:T30)
            n83 = To Variant(anything=w413) -> (Variant=w412:variant)
            n84 = property class="Slide"(reference=w419, error in=w417, "Value"=w412, "DisabledEnum"=T28."Disabled and Grayed Out" ("Disabled"), "Scale.Minimum"=0.0 ("Scale.Range:Minimum"), "Scale.Maximum"=60.0 ("Scale.Range:Maximum"), "Scale.RngStart"=0.0 ("Scale.Range:Start")) -> (error out=w416:errorcluster, "DigDisps[]"=w406:refnum<vi>[])  [unwired: 1 out]
            n85 = for {
              tunnel: w406 -> [w423] mode=indexing
              n86 = property class="DigNum"(reference=w423, "Visible"=FALSE) -> ()  [unwired: 1 in, 2 out]
            }
          }
          frame "By Zone stim. setup" {
            w429 = refnum<vi> refnum  # RadioButtonsControl
            n87 = To More Specific Class(target class=w429, reference=w430, error in=w427) -> (specific class reference=w428:refnum<vi>, error out=w426:errorcluster)
            n88 = property class="RadioBtnsControl"(reference=w428, error in=w426, "DisabledEnum"=T28."Disabled and Grayed Out" ("Disabled")) -> (error out=w425:errorcluster)  [unwired: 1 out]
          }
          frame "Reward and stimulation" {
            n89 = property class="Ctl"(reference=w433, error in=w432, "DisabledEnum"=T28."Disabled and Grayed Out" ("Disabled")) -> (error out=w431:errorcluster)  [unwired: 1 out]
          }
        }
        n90 = Build Array(w195, w200) -> (w199:string[])
      }
      "Controls references params" <- w35
      n91 = for {
        tunnel: w37 -> [w106] mode=indexing
        tunnel: [w96] -> w36 mode=indexing
        tunnel: w30 -> [w104]
        tunnel: [w100] -> w29 mode=indexing
        tunnel: w22 -> [w99]
        tunnel: w10 -> [w95]
        w108 = refnum<vi> refnum  # LVObjectRefNum
        n92 = To More Specific Class(target class=w108, reference=w106) -> (specific class reference=w109:refnum<vi>)  [unwired: 1 in, 1 out]
        n93 = property class="LVObjRef"(reference=w109, error in=w104) -> (error out=w103:errorcluster, "Value"=w107:variant)  [unwired: 1 out]
        n94 = Variant To Data(error in=w103, type=w106, Variant=w107) -> (data=w105:refnum<vi>, error out=w102:errorcluster)
        n95 = property class="Ctl"(reference=w105, error in=w102) -> (error out=w101:errorcluster, "Label.Text"=w98:string, "ClassName"=w97:string)  [unwired: 1 out]
        n96 = case "Indicators" shown="\"Diagram\"" w98 {
          selector: w98 -> [w110 _ _ _ _ _ _ _ _ _ _ _ _ _ _ _ _ _ _]
          tunnel: w105 -> [_ w124 w128 w130 w135 w139 _ _ _ _ w150 w155 w160 w165 w170 w175 w182 w189 _]
          tunnel: w101 -> [w113 w123 w127 w131 w136 w140 w142 w143 w144 w145 w149 w154 w159 w164 w169 w174 w181 w185 w191]
          tunnel: [w112 w122 w126 w133 w137 w141 w142 w143 w144 w145 w148 w153 w158 w163 w168 w173 w177 w188 w191] -> w100
          tunnel: w99 -> [_ _ _ w132 _ _ _ _ _ _ _ _ _ _ _ _ _ _ _]
          tunnel: w95 -> [_ _ _ _ _ _ _ _ _ _ _ _ _ _ _ _ w176 _ _]
          frame "", Default {
            n97 = xnode "Error Ring"("parameter 0"=w110) -> ("error out"=w111:errorcluster)
            n98 = Merge Errors(w113, w111) -> (w112:errorcluster)
          }
          frame "Cage size", "HW info", "Port" {
            n99 = property class="Ctl"(reference=w124, error in=w123, "Value"="") -> (error out=w122:errorcluster)  [unwired: 1 out]
          }
          frame "Ready" {
            n100 = property class="Ctl"(reference=w128, error in=w127, "Value"=FALSE) -> (error out=w126:errorcluster)  [unwired: 1 out]
          }
          frame "IO status" {
            n101 = call "SW_Get_Ports_IO_and_Inv_config.vi"("IO parameters cluster input"=w132) -> ("IO status indicator 2"=w129:T31)  [unwired: 4 out]
            n102 = property class="Ctl"(reference=w130, error in=w131, "Value"=w129) -> (error out=w133:errorcluster)  [unwired: 1 out]
          }
          frame "Ports Activity" {
            n103 = property class="Ctl"(reference=w135, error in=w136, "Value"=T26 {"IO1 act"=FALSE, "IO2 act"=FALSE, "IO3 act"=FALSE, "IO4 act"=FALSE} ("Ports Activity")) -> (error out=w137:errorcluster)  [unwired: 1 out]
          }
          frame "Active rules" {
            n104 = property class="Ctl"(reference=w139, error in=w140, "Value"=T27 {"01"=FALSE, "02"=FALSE, "03"=FALSE, "04"=FALSE, "05"=FALSE, "06"=FALSE, "07"=FALSE, "08"=FALSE, "09"=FALSE} ("Active rules")) -> (error out=w141:errorcluster)  [unwired: 1 out]
          }
          frame "Current Time" {
          }
          frame "Key_pressed" {
          }
          frame "Status" {
          }
          frame "Status History" {
          }
          frame "Since track start" {
            n105 = property class="Ctl"(reference=w150, error in=w149, "Value"=0.0, "DisabledEnum"=T28."Disabled and Grayed Out" ("Disabled")) -> (error out=w148:errorcluster)  [unwired: 1 out]
          }
          frame "Mouse speed" {
            n106 = property class="Ctl"(reference=w155, error in=w154, "Value"=waveform(dbl)[] [] ("History Data"), "DisabledEnum"=T28."Disabled and Grayed Out" ("Disabled")) -> (error out=w153:errorcluster)  [unwired: 1 out]
          }
          frame "Mouse speed, mm/s" {
            n107 = property class="Ctl"(reference=w160, error in=w159, "Value"=0.0, "DisabledEnum"=T28."Disabled and Grayed Out" ("Disabled")) -> (error out=w158:errorcluster)  [unwired: 1 out]
          }
          frame "Average speed, mm/s" {
            n108 = property class="Ctl"(reference=w165, error in=w164, "Value"=0.0, "DisabledEnum"=T28."Disabled and Grayed Out" ("Disabled")) -> (error out=w163:errorcluster)  [unwired: 1 out]
          }
          frame "CPU load" {
            n109 = property class="Ctl"(reference=w170, error in=w169, "Value"=0.0, "DisabledEnum"=T28."Disabled and Grayed Out" ("Disabled")) -> (error out=w168:errorcluster)  [unwired: 1 out]
          }
          frame "Run distance, m", "Running, perc. of time" {
            n110 = property class="Ctl"(reference=w175, error in=w174, "Value"=0.0, "DisabledEnum"=T28."Disabled and Grayed Out" ("Disabled")) -> (error out=w173:errorcluster)  [unwired: 1 out]
          }
          frame "Current zone" {
            w180 = refnum<vi> refnum  # Cluster
            n111 = To More Specific Class(target class=w180, reference=w182, error in=w181) -> (specific class reference=w178:refnum<vi>, error out=w179:errorcluster)
            n112 = call "UI_update_Zone_indicator_params_(univ).vi"("error in (no error)"=w179, "Geometry"=w176, "Zone indicator ref. in"=w178) -> ("error out"=w177:errorcluster)  [unwired: 7 in, 1 out]
          }
          frame "Histograms" {
            w186 = refnum<vi> refnum  # XYGraph
            n113 = disable-structure shown="Disabled" {
              frame Disabled {
                n114 = Unbundle By Name("Histogram initialization cluster") -> ()  [unwired: 9 out]
              }
              frame Enabled {
              }
            }
            n115 = To More Specific Class(target class=w186, reference=w189, error in=w185) -> (specific class reference=w187:refnum<vi>, error out=w184:errorcluster)
            n116 = property class="XYGraph"(reference=w187, error in=w184, "DisabledEnum"=T28."Disabled and Grayed Out" ("Disabled")) -> (error out=w188:errorcluster)  [unwired: 1 out]
          }
          frame "Diagram" {
          }
        }
        n117 = Build Array(w98, w97) -> (w96:string[])
      }
      "Indicators references params" <- w36
      n118 = Merge Errors(w13) -> (w12:errorcluster)
      n119 = Merge Errors(w12, w23, w29) -> (w28:errorcluster)
      n120 = property class="Pnl"(reference=w26, error in=w28, "DeferPanUpdts"=FALSE ("Defer Panel Updates")) -> (error out=w24:errorcluster)  [unwired: 1 out]
    }
    frame Error {
    }
  }
  "error out" <- w2
